vi "DC_Overvoltage_v2.vi"(4 "Polarity":enum16{"Positive", "Negative"}(ring), 5 "Write Task":string="BONTS-93-DC_Link_Input", 6 "# of Channels In":enum16{"1", "2"}(ring), 7 "Read Task":string="BONTS-93-DC_OV_Feedback", 8 "error in":errorcluster, 10 "Latch High Threshold":dbl=3.0, 11 "Latch Low Threshold":dbl=0.2) -> (0 "error out":errorcluster, 3 "Result":dbl[](array[numeric]))   [LabVIEW 2021]
uses:
  <vilib>/DAQmx/write.llb/DAQmx Write (Analog 1D DBL NChan 1Samp).vi
  <vilib>/DAQmx/read.llb/DAQmx Read (Analog DBL 1Chan 1Samp).vi
  <vilib>/DAQmx/miscellaneous.llb/DAQmx Fill In Error Info.vi
panel:
  in  "Starting Voltage":dbl=4.0
  out "VDC Unlatch":dbl[](array[numeric])
  out "V_Fault Unlatch":dbl format="%0.2f"
  out "V_Fault Latch":dbl format="%0.2f"
  in  "Max Voltage":dbl=5.2
  out "VDC Latch":dbl[](array[numeric])
  in  "Increments":i32=1000
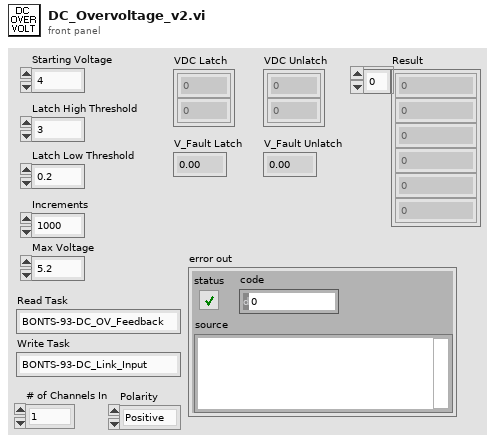
[diagram p1: front panel]
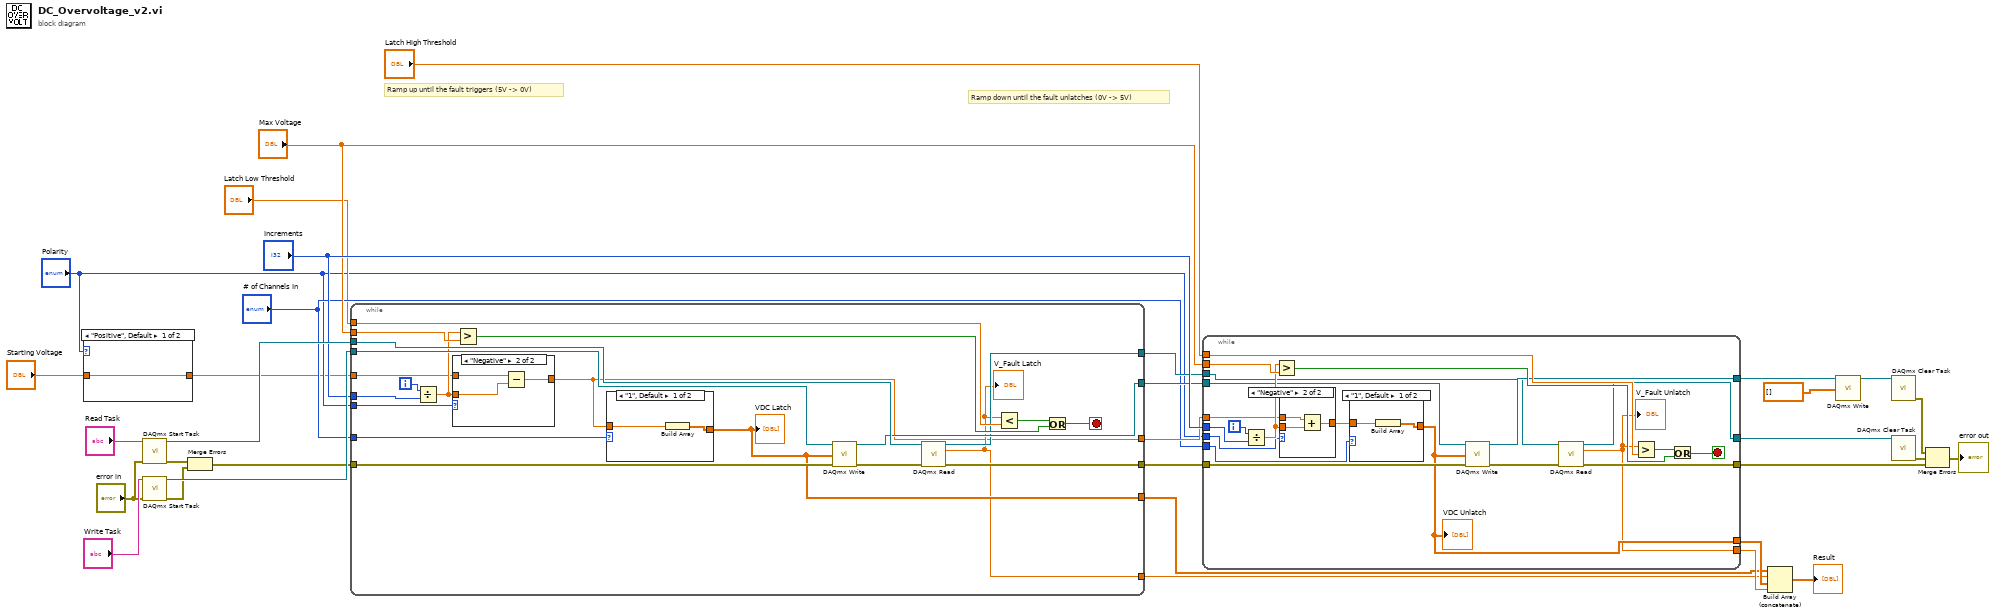
[diagram p0: block diagram]
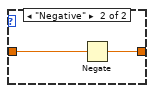
[diagram p2: hidden frame]
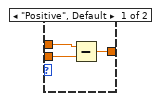
[diagram p3: hidden frame]
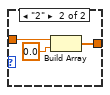
[diagram p4: hidden frame]
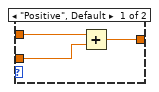
[diagram p5: hidden frame]
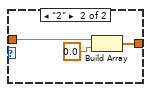
[diagram p6: hidden frame]
diagram:
  # "Ramp down until the fault unlatches (0V -> 5V)"
  # "Ramp up until the fault triggers (5V -> 0V)"
  n1 = case shown="\"Positive\", Default" "Polarity" {
    tunnel: "Starting Voltage" -> [w34 w36]
    tunnel: [w34 w35] -> w1
    frame "Positive", Default {
    }
    frame "Negative" {
      n2 = Negate(x=w36) -> (-x=w35:dbl)
    }
  }
  n3 = call <vilib>:"DAQmx Start Task.vi"("task/channels in"="Read Task", "error in"="error in") -> ("task out"=w30:refnum<k21>, "error out"=w21:errorcluster)  [unwired: 12 in]
  n4 = call <vilib>:"DAQmx Start Task.vi"("task/channels in"="Write Task", "error in"="error in") -> ("task out"=w32:refnum<k21>, "error out"=w20:errorcluster)  [unwired: 12 in]
  n5 = Merge Errors(w21, w20) -> (w22:errorcluster)
  n6 = while {
    tunnel: w30 -> [w57]
    tunnel: w32 -> [w56]
    tunnel: w22 -> [w55]
    tunnel: [w54] -> w18
    tunnel: "Latch Low Threshold" -> [w52]
    tunnel: "Increments" -> [w50]
    tunnel: "Max Voltage" -> [w49]
    tunnel: [w45] -> w17
    tunnel: [w44] -> w16
    tunnel: [w40] -> w15
    tunnel: [w43] -> w11
    tunnel: [w42] -> w12
    tunnel: w1 -> [w39]
    tunnel: "# of Channels In" -> [w38]
    tunnel: "Polarity" -> [w37]
    i -> [w51]
    stop <- w46 stop-if-true
    n7 = Divide(x=w51, y=w50) -> (x/y=w41:dbl)
    n8 = case shown="\"Negative\"" w37 {
      tunnel: w41 -> [w59 w63]
      tunnel: [w58 w62] -> w40
      tunnel: w39 -> [w60 w61]
      frame "Positive", Default {
        n9 = Add(x=w60, y=w59) -> (x+y=w58:dbl)
      }
      frame "Negative" {
        n10 = Subtract(x=w61, y=w63) -> (x-y=w62:dbl)
      }
    }
    n11 = Greater?(x=w41, y=w49) -> (0:w47:bool)
    n12 = case shown="\"1\", Default" w38 {
      tunnel: [w65 w67] -> w43
      tunnel: w40 -> [w64 w66]
      frame "1", Default {
        n13 = Build Array(w64) -> (w65:dbl[])
      }
      frame "2" {
        n14 = Build Array(w66, 0.0 ("element")) -> (w67:dbl[])
      }
    }
    "VDC Latch" <- w43
    n15 = call-poly <vilib>:"DAQmx Write.vi"("task/channels in"=w56, "data"=w43, "error in"=w55) -> ("task out"=w45:refnum<k21>, "error out"=w53:errorcluster)  [unwired: 10 in, 1 out]
    n16 = call-poly <vilib>:"DAQmx Read.vi"("task/channels in"=w57, "error in"=w53) -> ("task out"=w44:refnum<k21>, "data"=w42:dbl, "error out"=w54:errorcluster)  [unwired: 11 in]
    "V_Fault Latch" <- w42
    n17 = Less?(x=w42, y=w52) -> (x < y?=w48:bool)
    n18 = Or(x=w48, y=w47) -> (x .or. y?=w46:bool)
  }
  n19 = while {
    tunnel: [w89] -> w24
    tunnel: "Latch High Threshold" -> [w87]
    tunnel: "Increments" -> [w85]
    tunnel: "Max Voltage" -> [w84]
    tunnel: [w80] -> w27
    tunnel: [w79] -> w9
    tunnel: w18 -> [w78]
    tunnel: w15 -> [w75]
    tunnel: w17 -> [w74]
    tunnel: w16 -> [w73]
    tunnel: [w72] -> w13
    tunnel: [w71] -> w14
    tunnel: "# of Channels In" -> [w70]
    tunnel: "Polarity" -> [w69]
    i -> [w86]
    stop <- w81 stop-if-true
    n20 = Divide(x=w86, y=w85) -> (x/y=w76:dbl)
    n21 = Greater?(x=w76, y=w84) -> (0:w82:bool)
    n22 = case shown="\"Negative\"" w69 {
      tunnel: [w92 w93] -> w77
      tunnel: w76 -> [w90 w94]
      tunnel: w75 -> [w91 w95]
      frame "Positive", Default {
        n23 = Subtract(x=w91, y=w90) -> (x-y=w92:dbl)
      }
      frame "Negative" {
        n24 = Add(x=w95, y=w94) -> (x+y=w93:dbl)
      }
    }
    n25 = case shown="\"1\", Default" w70 {
      tunnel: w77 -> [w96 w99]
      tunnel: [w97 w98] -> w72
      frame "1", Default {
        n26 = Build Array(w96) -> (w97:dbl[])
      }
      frame "2" {
        n27 = Build Array(w99, 0.0 ("element")) -> (w98:dbl[])
      }
    }
    "VDC Unlatch" <- w72
    n28 = call-poly <vilib>:"DAQmx Write.vi"("task/channels in"=w74, "data"=w72, "error in"=w78) -> ("task out"=w79:refnum<k21>, "error out"=w88:errorcluster)  [unwired: 10 in, 1 out]
    n29 = call-poly <vilib>:"DAQmx Read.vi"("task/channels in"=w73, "error in"=w88) -> ("task out"=w80:refnum<k21>, "data"=w71:dbl, "error out"=w89:errorcluster)  [unwired: 11 in]
    "V_Fault Unlatch" <- w71
    n30 = Greater?(x=w71, y=w87) -> (0:w83:bool)
    n31 = Or(x=w83, y=w82) -> (x .or. y?=w81:bool)
  }
  n32 = Build Array (concatenate)(w11, w12, w13, w14) -> (→"Result":dbl[])
  n33 = call-poly <vilib>:"DAQmx Write.vi"("task/channels in"=w9, "data"=dbl[] []) -> ("task out"=w8:refnum<k21>)  [unwired: 11 in, 2 out]
  n34 = call <vilib>:"DAQmx Clear Task.vi"("task in"=w8) -> ("error out"=w26:errorcluster)  [unwired: 14 in]
  n35 = call <vilib>:"DAQmx Clear Task.vi"("task in"=w27) -> ("error out"=w25:errorcluster)  [unwired: 14 in]
  n36 = Merge Errors(w26, w25, w24) -> (→"error out":errorcluster)
